vi "Framework Configuration 1.1 Initialize.vi"(8 "error in (no error)":errorcluster, 9 "dsf version":T2, 10 "json version":T2, 11 "dsf configuration json":string) -> (0 "error out":errorcluster, 3 "framework configuration 1.1":T1)   [LabVIEW 2017, in "DSF Core.lvlib" / "Configuration Session.lvclass"]
uses:
  Configuration Session.lvclass
  Typedefs/DSF Version Info.ctl
  Framework Configuration 1.1.ctl
  DSF Core.lvlib
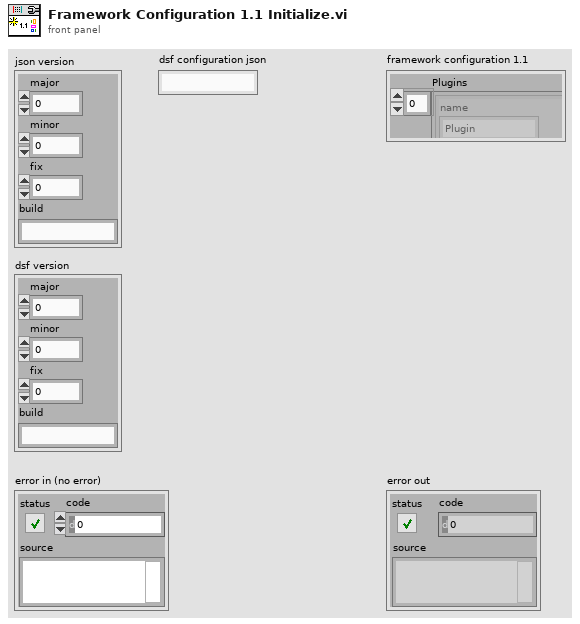
[diagram p1: front panel]
types:
  T1 = typedef "DSF Core.lvlib/Configuration Session.lvclass/Framework Configuration 1.1.ctl" = cluster{"Plugins":cluster{"name":string, "components":string[], "cycle timing":cluster{"priority":u64, "decimation":u64, "offset":u64}, "threads":cluster{"buffer converter settings":cluster{"key":string, "value":string}[], "transceiver settings":cluster{"key":string, "value":string}[], "custom settings":cluster{"key":string, "value":string}[], "processor":i32, "priority offset":i16}[], "Transfer Groups":cluster{"name":string, "direction":enum8{"Tx", "Rx"}, "cycle timing":cluster{"priority":u64, "decimation":u64, "offset":u64}, "thread index":i32, "settings":cluster{"key":string, "value":string}[], "Transfers":cluster{"name":string, "byte order":enum8{"big-endian", "little-endian"}, "settings":cluster{"key":string, "value":string}[], "channels":cluster{"string offset":u64, "string data type":enum8{"Bool", "SGL", "DBL", "I8", "I16", "I32", "I64", "U8", "U16", "U32", "U64"}, "engine data type":enum8{"Bool", "SGL", "DBL", "I8", "I16", "I32", "I64", "U8", "U16", "U32", "U64"}, "name":string, "settings":cluster{"key":string, "value":string}[], "units":string}[]}[], "timeout behavior":enum8{"Increment Late Count", "Throw Error"}}[], "settings":cluster{"key":string, "value":string}[]}[]}
  T2 = typedef "DSF Core.lvlib/DSF Version Info.ctl" = cluster{"major":u32, "minor":u32, "fix":u32, "build":string}
  T3 = typedef "DSF Core.lvlib/Configuration Session.lvclass/Framework Configuration 1.0.ctl" = cluster{"Plugins":cluster{"name":string, "components":string[], "cycle timing":cluster{"priority":u64, "decimation":u64, "offset":u64}, "threads":cluster{"buffer converter settings":cluster{"key":string, "value":string}[], "transceiver settings":cluster{"key":string, "value":string}[], "custom settings":cluster{"key":string, "value":string}[], "processor":i32, "priority offset":i16}[], "Transfer Groups":cluster{"name":string, "direction":enum8{"Tx", "Rx"}, "cycle timing":cluster{"priority":u64, "decimation":u64, "offset":u64}, "thread index":i32, "settings":cluster{"key":string, "value":string}[], "Transfers":cluster{"name":string, "byte order":enum8{"big-endian", "little-endian"}, "settings":cluster{"key":string, "value":string}[], "channels":cluster{"string offset":u64, "string data type":enum8{"Bool", "SGL", "DBL", "I8", "I16", "I32", "I64", "U8", "U16", "U32", "U64"}, "engine data type":enum8{"Bool", "SGL", "DBL", "I8", "I16", "I32", "I64", "U8", "U16", "U32", "U64"}, "name":string, "settings":cluster{"key":string, "value":string}[], "units":string}[]}[], "timeout behavior":enum8{"Increment Late Count", "Throw Error"}}[], "settings":cluster{"key":string, "value":string}[]}[]}
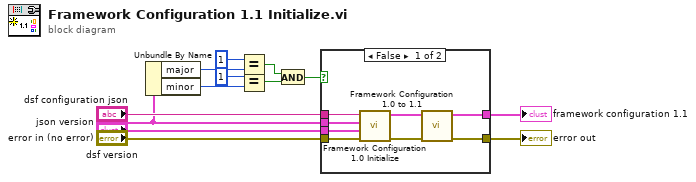
[diagram p0: block diagram]
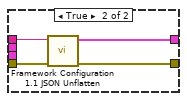
[diagram p2: hidden frame]
diagram:
  n1 = Unbundle By Name("json version") -> ("major"=w9:u32, "minor"=w12:u32)
  n2 = Equal?(x=u32 1, y=w9) -> (x = y?=w5:bool)
  n3 = Equal?(x=u32 1, y=w12) -> (x = y?=w6:bool)
  n4 = And(x=w5, y=w6) -> (x .and. y?=w4:bool)
  n5 = case shown="False" w4 {
    tunnel: "error in (no error)" -> [w20 w25]
    tunnel: "dsf configuration json" -> [w21 w24]
    tunnel: [w16 w23] -> w11
    tunnel: [w17 w22] -> w10
    tunnel: "json version" -> [w15 _]
    tunnel: "dsf version" -> [w14 _]
    frame False {
      n6 = call "Framework Configuration 1.0 Initialize.vi"("error in (no error)"=w20, "dsf version"=w14, "json version"=w15, "dsf configuration json"=w21) -> ("error out"=w19:errorcluster, "framework configuration 1.0"=w18:T3)  [unwired: 6 in]
      n7 = call "Framework Configuration 1.0 to 1.1.vi"("error in (no error)"=w19, "framework configuration 1.0"=w18) -> ("error out"=w17:errorcluster, "framework configuration 1.1"=w16:T1)  [unwired: 8 in]
    }
    frame True {
      n8 = call "Framework Configuration 1.1 JSON Unflatten.vi"("error in (no error)"=w25, "dsf configuration json"=w24) -> ("error out"=w22:errorcluster, "framework configuration 1.1"=w23:T1)  [unwired: 8 in]
    }
  }
  "error out" <- w10
  "framework configuration 1.1" <- w11
